vi "BigTiFF-test.vi"() -> ()   [LabVIEW 2011]
uses:
  TiffModules/ReadTiffPage_U16_text_res.vi
panel:
  out "Reading":i32
  out "TIFF file":T1 {"BigTiff,Endian" items=["Big-Endian"=0, "Native"=1, "Little-Endian"=2, "BigTiff-Big-Endian"=256, "Bigtiff,Native"=257, "Biftiff,Littleendian"=258]}
  out "Intensity Graph":u16[][](graph)
  in  "file path":path=path "\\\\till-server\\data/Entwicklung/FlumiasNo3/20220131_SIP-vieleraw/41_Single_SIM_488_Camera1/Image_I41_B1_SIM_488_Camera1_Raw.tif"
  # "seems to work, not RGB"
  # "first is 0"
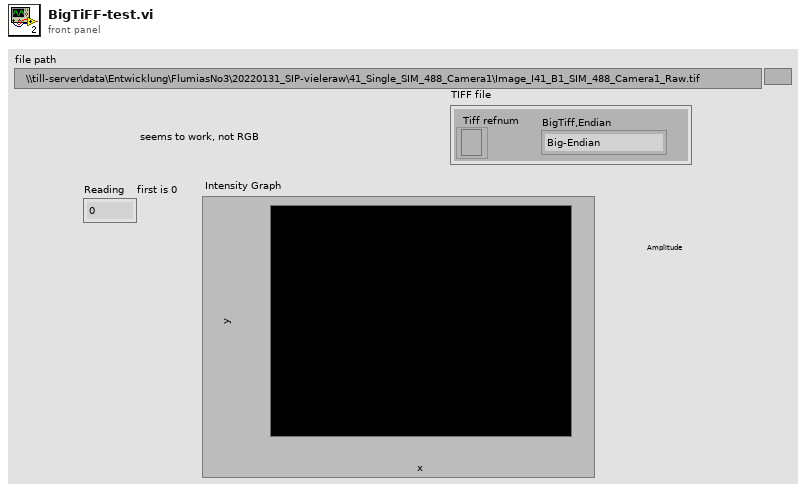
[diagram p1: front panel]
types:
  T1 = cluster{"Tiff refnum":refnum<file>, "BigTiff,Endian":u16}
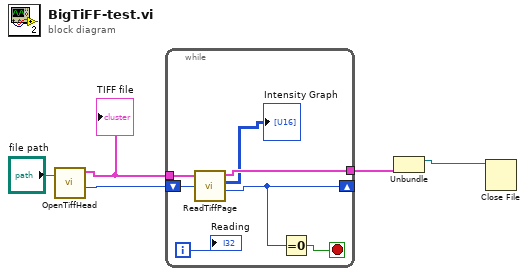
[diagram p0: block diagram]
diagram:
  n1 = call "OpenTiffHead.vi"("file path"="file path") -> ("TIFF file"=w3:T1, "first Diroffset"=w1:u64)  [unwired: 2 in, 1 out]
  "TIFF file" <- w3
  n2 = while {
    tunnel: w3 -> [w10]
    tunnel: [w8] -> w2
    shift-right: [w6] -> _
    shift-left: w1 -> [w9]
    i -> [w11]
    stop <- w12 stop-if-true
    n3 = call-poly "ReadTiffPage.vi"("TIFF file"=w10, "IFDoffset"=w9) -> ("TIFF file out"=w8:T1, "16-bit pixmap"=→"Intensity Graph":u16[][], "Next offset"=w6:i64)  [unwired: 3 in, 3 out]
    n4 = Equal To 0?(x=w6) -> (x = 0?=w12:bool)
    "Reading" <- w11
  }
  n5 = Unbundle(w2) -> ("Tiff refnum"=w4:refnum<file>)  [unwired: 1 out]
  n6 = Close File(refnum=w4) -> ()  [unwired: 1 in, 2 out]
